vi "Query_Olympus_wo_Login.vi"(8 "error in (no error)":errorcluster, 9 "Device Number\n(1: -Condensor\n     - Objective\n     - Lamp\n     - Shutter\n2: - Z-Motion\n   - Autofocus)":i32=1, 10 "String":string, 11 "VISA Resource Name In":refnum<visa-resource-name>) -> (0 "error out":errorcluster, 2 "Result":string, 3 "VISA Resource Name Out":refnum<visa-resource-name>)   [LabVIEW 2018]
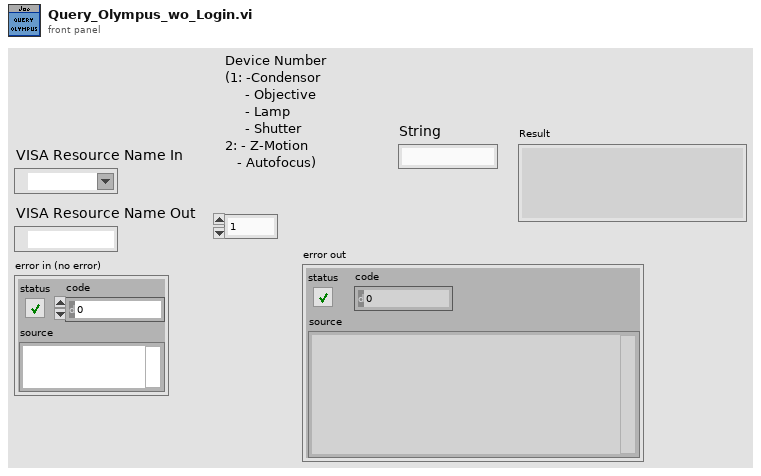
[diagram p1: front panel]
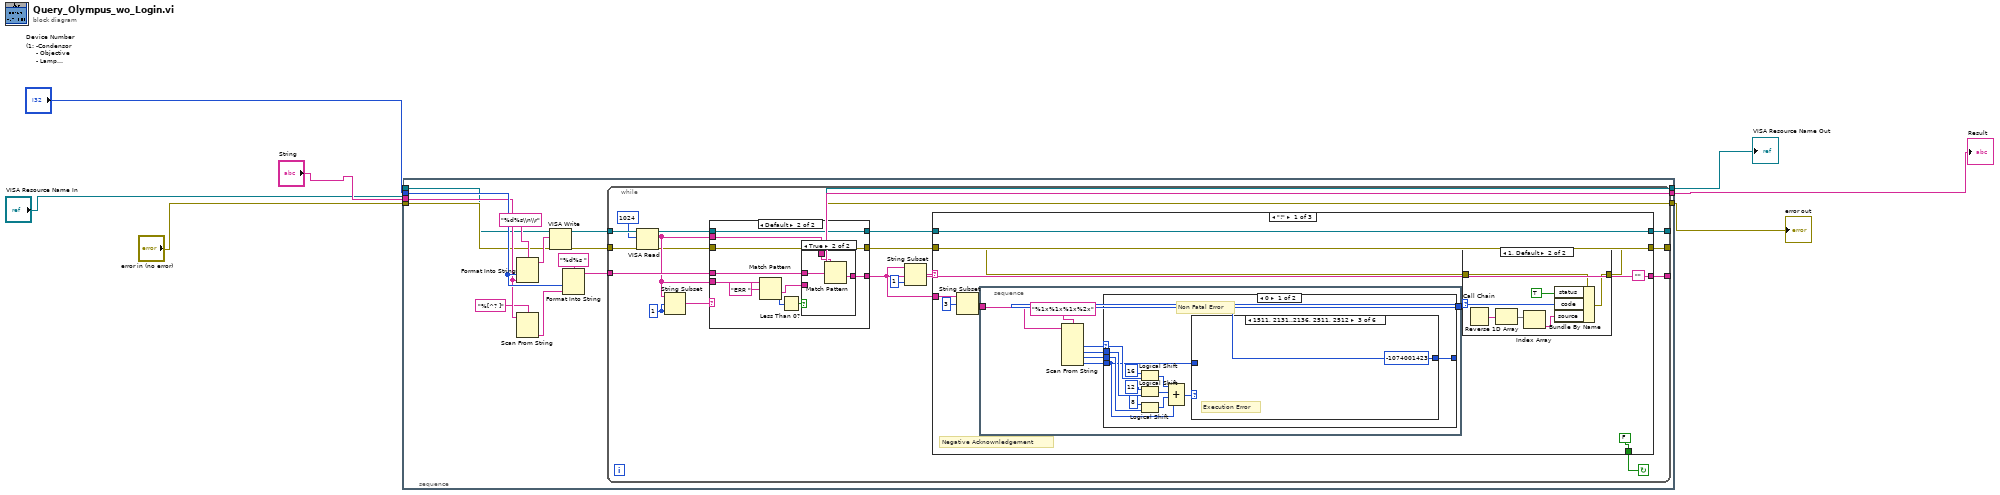
[diagram p0: block diagram]
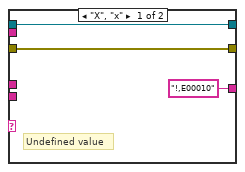
[diagram p2: hidden frame]
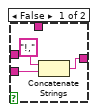
[diagram p3: hidden frame]
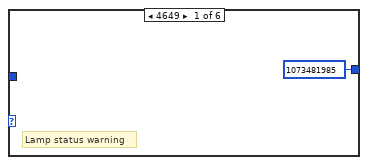
[diagram p4: hidden frame]
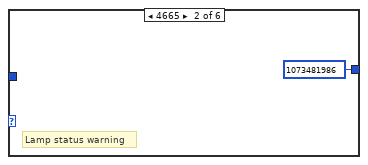
[diagram p5: hidden frame]
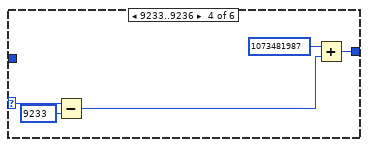
[diagram p6: hidden frame]
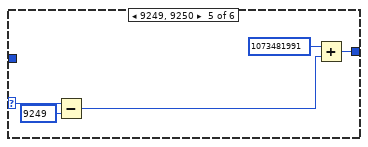
[diagram p7: hidden frame]
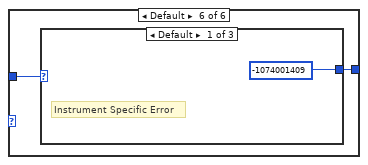
[diagram p8: hidden frame]
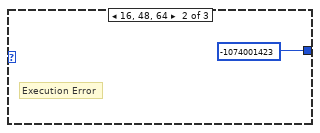
[diagram p9: hidden frame]
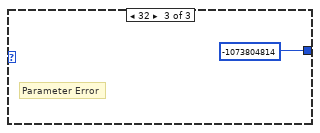
[diagram p10: hidden frame]
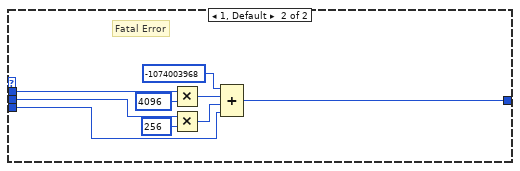
[diagram p11: hidden frame]
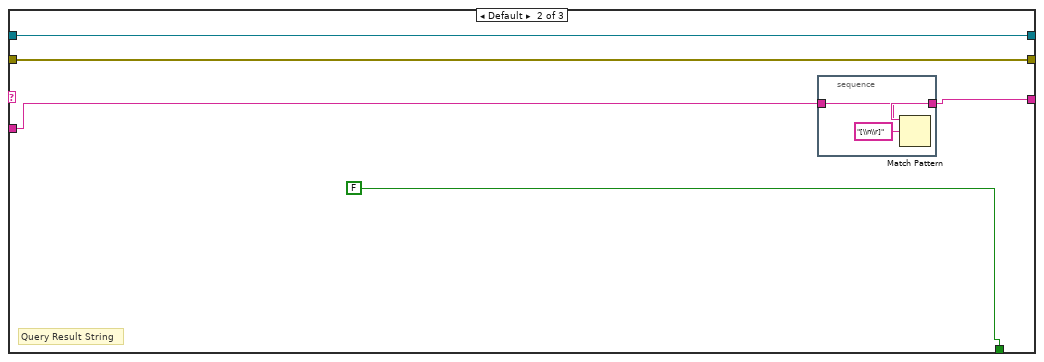
[diagram p13: hidden frame]
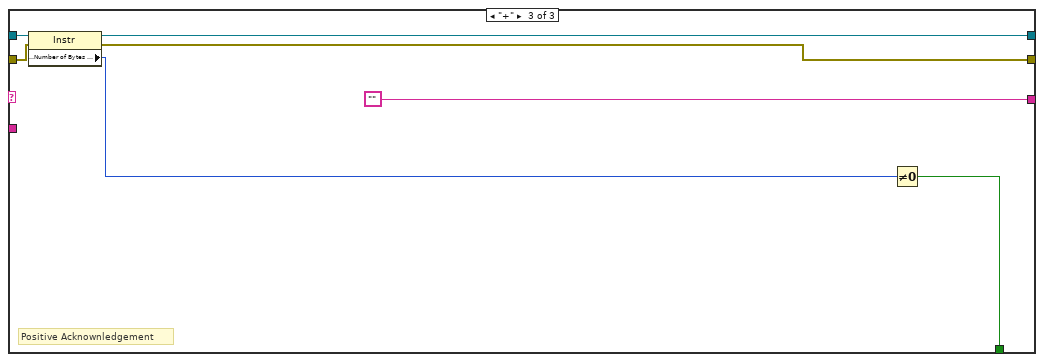
[diagram p14: hidden frame]
diagram:
  n1 = stacked-sequence {
    tunnel: [w20] -> w3
    tunnel: [w22] -> w7
    tunnel: [w21] -> w2
    tunnel: "error in (no error)" -> [w9]
    tunnel: "String" -> [w15]
    tunnel: "Device Number\n(1: -Condensor\n     - Objective\n     - Lamp\n     - Shutter\n2: - Z-Motion\n   - Autofocus)" -> [w16]
    tunnel: "VISA Resource Name In" -> [w8]
    frame #0 {
      n2 = Format Into String(format string="%d%s\\n\\r", w16, w15) -> (resulting string=w14:string)  [unwired: 2 in, 1 out]
      n3 = Scan From String(format string="%[^? ]", input string=w15) -> (output 1=w17:string)  [unwired: 3 in, 3 out]
      n4 = VISA Write(VISA resource name=w8, write buffer=w14, error in (no error)=w9) -> (VISA resource name out=w12:refnum<visa-resource-name>, error out=w11:errorcluster)  [unwired: 1 out]
      n5 = Format Into String(format string="%d%s ", w16, w17) -> (resulting string=w19:string)  [unwired: 2 in, 1 out]
      n6 = while {
        tunnel: w11 -> [w40]
        tunnel: w12 -> [w39]
        tunnel: w19 -> [w37]
        tunnel: [w36] -> w20
        tunnel: [w35] -> w21
        tunnel: [w34] -> w22
        stop <- w30 continue-if-true
        w29 = 1 ("length (rest)")
        n7 = VISA Read(VISA resource name=w39, byte count=u32 1024, error in (no error)=w40) -> (VISA resource name out=w26:refnum<visa-resource-name>, read buffer=w27:string, error out=w24:errorcluster)  [unwired: 1 out]
        n8 = String Subset(string=w27, offset (0)=w29, length (rest)=w29) -> (substring=w28:string)
        n9 = case shown="Default" w28 {
          tunnel: w37 -> [_ w53]
          tunnel: ["!,E00010" w52] -> w33
          tunnel: w27 -> [_ w47]
          tunnel: w27 -> [_ w46]
          tunnel: w26 -> [w43 w45]
          tunnel: [w43 w45] -> w25
          tunnel: w24 -> [w42 w44]
          tunnel: [w42 w44] -> w23
          frame "X", "x" {
            # "Undefined value"
          }
          frame Default {
            n10 = Match Pattern(string=w46, regular expression="ERR ") -> (after substring=w48:string, offset past match=w50:i32)  [unwired: 1 in, 2 out]
            n11 = Less Than 0?(x=w50) -> (x < 0?=w49:bool)
            n12 = case shown="True" w49 {
              tunnel: w53 -> [_ w59]
              tunnel: [w55 w58] -> w52
              tunnel: w47 -> [_ w57]
              tunnel: w48 -> [w56 _]
              frame False {
                n13 = Concatenate Strings("!," ("string"), w56) -> (w55:string)
              }
              frame True {
                n14 = Match Pattern(string=w57, regular expression=w59) -> (after substring=w58:string)  [unwired: 1 in, 3 out]
              }
            }
          }
        }
        n15 = String Subset(string=w33, length (rest)=1 ("length (rest)")) -> (substring=w32:string)  [unwired: 1 in]
        n16 = case shown="\"!\"" w32 {
          tunnel: w23 -> [w62 w127 w135]
          tunnel: [w61 w127 w133] -> w36
          tunnel: w23 -> [_ _ _]
          tunnel: [w67 w126 w134] -> w35
          tunnel: w25 -> [w67 w126 w136]
          tunnel: ["" w124 ""] -> w34
          tunnel: w33 -> [w66 w125 _]
          tunnel: [FALSE FALSE w131] -> w30
          frame "!" {
            # "Negative Acknownledgement"
            n17 = String Subset(string=w66, offset (0)=3) -> (substring=w64:string)  [unwired: 1 in]
            n18 = stacked-sequence {
              tunnel: [w75] -> w63
              tunnel: w64 -> [w70]
              frame #0 {
                n19 = Scan From String(format string="%1x%1x%1x%2x", input string=w70) -> (output 1=w71:u32, output 2=w72:u32, output 3=w73:u32, output 4=w74:u32)  [unwired: 6 in, 3 out]
                n20 = case shown="0" w71 {
                  selector: w71 -> [w85 _]
                  tunnel: w72 -> [w84 w113]
                  tunnel: w73 -> [w83 w112]
                  tunnel: w74 -> [w77 w107]
                  tunnel: [w87 w106] -> w75
                  frame 0 {
                    # "Non Fatal Error"
                    n21 = Logical Shift(y=16, x=w85) -> (x << y=w80:u32)
                    n22 = Logical Shift(y=12, x=w84) -> (x << y=w79:u32)
                    n23 = Logical Shift(y=8, x=w83) -> (x << y=w78:u32)
                    n24 = Compound Arithmetic op=ADD(w80, w79, w78, w77) -> (w76:u32)
                    n25 = case shown="1511, 2131..2136, 2511, 2512" w76 {
                      selector: w76 -> [_ _ _ w95 w100 _]
                      tunnel: [1073481985 1073481986 -1074001423 w93 w98 w102] -> w87
                      tunnel: w77 -> [_ _ _ _ _ w101]
                      frame 4649 {
                        # "Lamp status warning"
                      }
                      frame 4665 {
                        # "Lamp status warning"
                      }
                      frame 5393, 8497..8502, 9489, 9490 {
                        # "Execution Error"
                      }
                      frame 9233..9236 {
                        n26 = Subtract(x=w95, y=9233) -> (x-y=w91:u32)
                        n27 = Add(x=1073481987, y=w91) -> (x+y=w93:u32)
                      }
                      frame 9249, 9250 {
                        n28 = Subtract(x=w100, y=9249) -> (x-y=w96:u32)
                        n29 = Add(x=1073481991, y=w96) -> (x+y=w98:u32)
                      }
                      frame Default {
                        n30 = case shown="Default" w101 {
                          tunnel: [-1074001409 -1074001423 -1073804814] -> w102
                          frame Default {
                            # "Instrument Specific Error"
                          }
                          frame 16, 48, 64 {
                            # "Execution Error"
                          }
                          frame 32 {
                            # "Parameter Error"
                          }
                        }
                      }
                    }
                  }
                  frame 1, Default {
                    # "Fatal Error"
                    n31 = Multiply(x=w113, y=4096) -> (x*y=w109:u32)
                    n32 = Multiply(x=w112, y=256) -> (x*y=w108:u32)
                    n33 = Compound Arithmetic op=ADD(-1074003968, w109, w108, w107) -> (w106:u32)
                  }
                }
              }
            }
            n34 = case shown="1, Default" w63 {
              selector: w63 -> [_ w119]
              tunnel: w62 -> [w115 w120]
              tunnel: [w115 w116] -> w61
              frame 0 {
              }
              frame 1, Default {
                n35 = Call Chain() -> (call chain=w122:string[])
                n36 = Reverse 1D Array(array=w122) -> (reversed array=w121:string[])
                n37 = Index Array(array=w121) -> (element=w118:string)  [unwired: 1 in]
                n38 = Bundle By Name(cluster=w120, "status"=TRUE, "code"=w119, "source"=w118) -> (w116:errorcluster)
              }
            }
          }
          frame Default {
            # "Query Result String"
            n39 = stacked-sequence {
              tunnel: [w130] -> w124
              tunnel: w125 -> [w128]
              frame #0 {
                n40 = Match Pattern(string=w128, regular expression="[\\n\\r]") -> (before substring=w130:string)  [unwired: 1 in, 3 out]
              }
            }
          }
          frame "+" {
            # "Positive Acknownledgement"
            n41 = property class="Instr"(reference=w136, error in=w135) -> (reference out=w134:refnum<visa-resource-name>, error out=w133:errorcluster, "Serial Settings:Number of Bytes at Serial Port"=w132:u32)
            n42 = Not Equal To 0?(x=w132) -> (x != 0?=w131:bool)
          }
        }
      }
    }
  }
  "error out" <- w3
  "Result" <- w7
  "VISA Resource Name Out" <- w2
